vi "IMAQ Detect Rectangles.vi"(4 "Minimum match score":dbl, 6 "Curve Parameters":T5={"Extraction Mode"=0, "Edge Threshold"=75, "Edge Filter Size"=1, "Min Length"=25, "Row Search Step Size"=15, "Col Search Step Size"=15, "Max Endpoint Gap"=10, "Closed"=FALSE, "Subpixel"=FALSE} {"Max Endpoint Gap" min=0; "Col Search Step Size" min=1 max=255 step=1; "Row Search Step Size" min=1 max=255 step=1; "Min Length" min=0; "Edge Filter Size" items=["Fine", "Normal", "Controur Tracing"]; "Edge Threshold" min=1 max=65535 step=1; "Extraction Mode" items=["Normal", "Uniform Regions"]}, 7 "ROI Descriptor":T7 {"Contours"."Type" items=["No Selection", "Point", "Line", "Rectangle", "Oval", "Polygon", "Freehand Region", "Annulus", "Unused2", "Unused3", "Broken Line", "Freehand Line", "Rotated Rectangle"]}, 8 "error in (no error)":errorcluster, 9 "Match Options":T3 {"Range Settings"."Match Constraints" items=["Rotation Angle (degrees)", "Scale Factor (%)", "Occlusion (%)"]}, 10 "Rectangle Descriptor":T2={"Min Width"=10.0, "Max Width"=200.0, "Min Height"=10.0, "Max Height"=100.0}, 11 "Image":T6) -> (0 "error out":errorcluster, 2 "Number of Matches Returned":i32, 3 "Rectangles":T1(array[cluster]) {"Corners"."Y" format="%.2f"; "Corners"."X" format="%.2f"})   [LabVIEW 2025, in "NI_Vision_Development_Module.lvlib"]
doc: "Searches for rectangles in an image."
uses:
  <vilib>/vision/NI_Vision_Development_Module.lvlib
  <vilib>/vision/Image Controls.llb/IMAQ Image.ctl
  <vilib>/vision/Pattern Matching.llb/IMAQ Curve Parameters.ctl
  <vilib>/vision/Shape Detection.llb/ShapeDetectionMatchOptions.ctl
  <vilib>/vision/Pattern Matching.llb/IMAQ Match Range Setting.ctl
  nivision.dll
panel:
  # "Range"
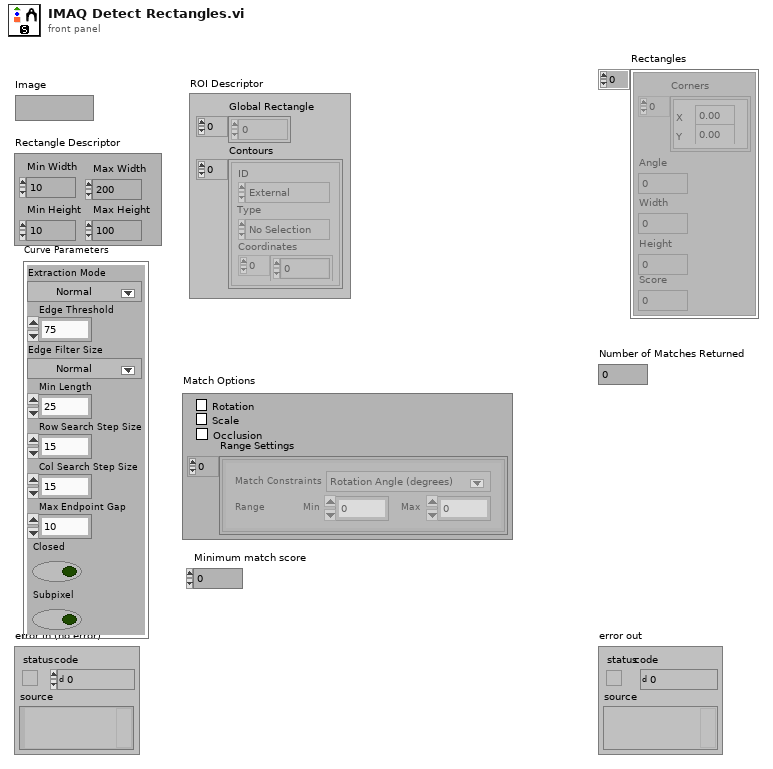
[diagram p1: front panel]
types:
  T1 = cluster{"Corners":cluster{"X":sgl, "Y":sgl}[], "Angle":dbl, "Width":dbl, "Height":dbl, "Score":dbl}[]
  T2 = cluster{"Min Width":dbl, "Max Width":dbl, "Min Height":dbl, "Max Height":dbl}
  T3 = typedef "ShapeDetectionMatchOptions.ctl" = cluster{"Rotation":bool, "Scale":bool, "Occlusion":bool, "Range Settings":T4[]}
  T4 = typedef "IMAQ Match Range Setting.ctl" = cluster{"Match Constraints":u32, "Min":dbl, "Max":dbl}
  T5 = typedef "IMAQ Curve Parameters.ctl" = cluster{"Extraction Mode":u32, "Edge Threshold":i32, "Edge Filter Size":u32, "Min Length":i32, "Row Search Step Size":i32, "Col Search Step Size":i32, "Max Endpoint Gap":i32, "Closed":bool, "Subpixel":bool}
  T6 = typedef "IMAQ Image.ctl" = refnum<image>
  T7 = cluster{"Global Rectangle":i32[], "Contours":cluster{"ID":enum32{"External", "Internal"}, "Type":u32, "Coordinates":i32[]}[]}
  T8 = cluster{"Corners":cluster{"X":sgl, "Y":sgl}[], "Orientation (degrees)":dbl, "Width":dbl, "Height":dbl, "Score":dbl}[]
  T9 = typedef "IMAQ Curve Parameters Internal.ctl" = cluster{"Extraction Mode":u32, "Edge Threshold":i32, "Edge Filter Size":u32, "Min Length":i32, "Row Search Step Size":i32, "Col Search Step Size":i32, "Max Endpoint Gap":i32, "Closed":i32, "Subpixel":i32}
  T10 = cluster{"Rotation":i32, "Scale":i32, "Occlusion":i32, "Array":T4[]}
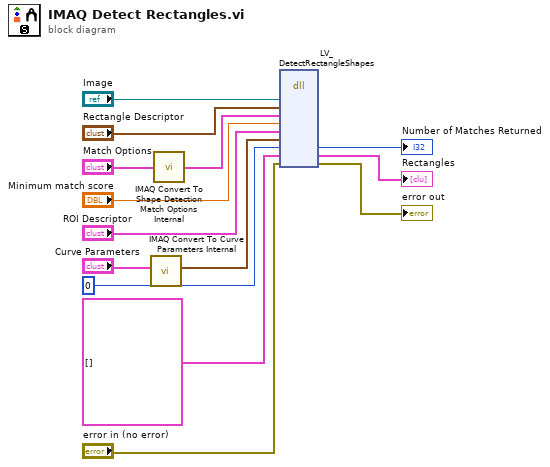
[diagram p0: block diagram]
diagram:
  n1 = call "IMAQ Convert To Curve Parameters Internal"("Curve Parameters"="Curve Parameters") -> ("Curve Parameters (internal)"=w1:T9)  [unwired: 10 out]
  n2 = call "IMAQ Convert To Shape Detection Match Options Internal"("Match Options In"="Match Options") -> ("Match Options Out"=w3:T10)
  n3 = dll-call lib="nivision.*" fn="LV_DetectRectangleShapes"("image"="Image", "rectangleDescriptor"="Rectangle Descriptor", "shapeDetectionOptions"=w3, "minimumMatchScore"="Minimum match score", "roi"="ROI Descriptor", "curveParameters"=w1, "nMatchesFound"=0 ("Number of Matches Returned"), "matchReport"=T8 [] ("Rectangles"), "cluster"="error in (no error)") -> ("nMatchesFound"=→"Number of Matches Returned":i32, "matchReport"=→"Rectangles":T8, "cluster"=→"error out":errorcluster)  [unwired: 9 in, 3 out]
